vi "Get NEC Message.vi"(8 "error in (no error)":errorcluster) -> (0 "error out":errorcluster, 5 "Message":string)   [LabVIEW 2016, in "Stream Error.lvlib" / "Error Interface.lvclass"]
doc: "--\nCopyright © 2017 Composed SystemsI All rights reserved.\n\nAuthor: Jon McBee <jon.mcbee@composed.io>\n\nThis library is provided \"AS IS\" ,WITHOUT WARRANTIES OR\nCONDITIONS OF ANY KIND, either express or implied.\n\nComposed Systems -- composed.io\n\nStream 0.0.1.1\nJon McBee - Composed Systems\nCopyright (c) 2017, Composed Systems"
uses:
  <userlib>/Composed Systems/Stream/Error/Classes/Error Interface/Error Interface.lvclass
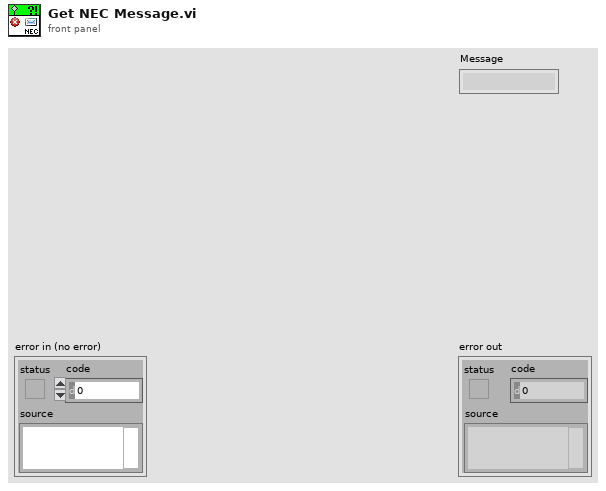
[diagram p1: front panel]
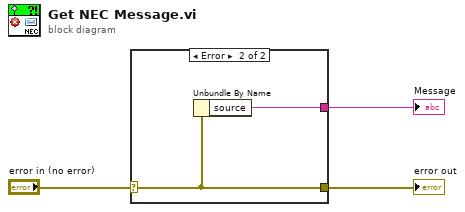
[diagram p0: block diagram]
diagram:
  n1 = case shown="Error" "error in (no error)" {
    selector: "error in (no error)" -> [w4 w6]
    tunnel: [w4 w6] -> w2
    tunnel: [_ w5] -> w1
    frame No Error {
    }
    frame Error {
      n2 = Unbundle By Name(w6) -> ("source"=w5:string)
    }
  }
  "error out" <- w2
  "Message" <- w1
